vi "SWaT pump flow.vi"(4 "State":i16, 5 "Time":dbl format="%.2f", 6 "Sensor Values":dbl[](array[numeric]), 7 "Set Points":dbl[](array[numeric])) -> (0 "required data":T1={"Set Point names"=["L Tube Settler (mm)", "D Tube Settler (mm)", "Tube angle (degrees)", "Capture Velocity (mm/s)", ""], "required number of setpoints"=4, "required number of sensors"=0, "Sensor names"=[]}, 3 "output value":dbl)   [LabVIEW 2019]
panel:
  # "Enter the correct information for this control code in the required data structure below. Then make the current value default by right clicking on the border of the data structure."
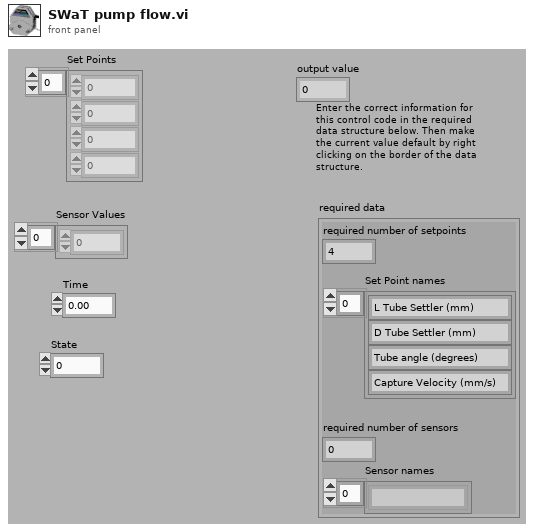
[diagram p1: front panel]
types:
  T1 = cluster{"Set Point names":string[], "required number of setpoints":u8, "required number of sensors":u8, "Sensor names":string[]}
  T2 = cluster{"Set Points[0]":dbl, "Set Points[1]":dbl, "Set Points[2]":dbl, "Set Points[3]":dbl, "Set Points[4]":dbl}
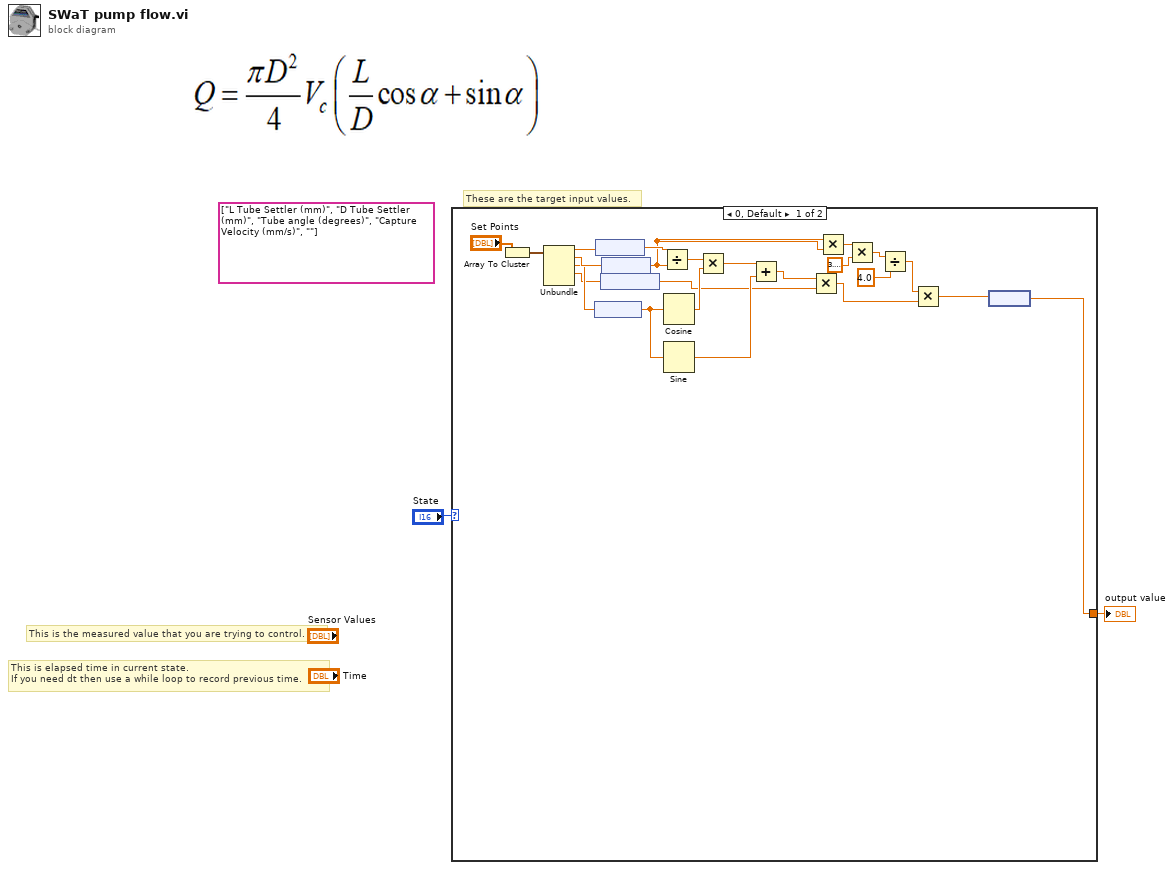
[diagram p0: block diagram]
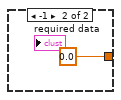
[diagram p2: hidden frame]
diagram:
  (unwired) string[] ["L Tube Settler (mm)", "D Tube Settler (mm)", "Tube angle (degrees)", "Capture Velocity (mm/s)", ""] ("Set Point names")
  # "These are the target input values."
  # "This is the measured value that you are trying to control."
  # "This is elapsed time in current state.\nIf you need dt then use a while loop to record previous time."
  n1 = case shown="0, Default" "State" {
    tunnel: [w7 0.0 ("fraction on")] -> w1
    frame 0, Default {
      n2 = Array To Cluster(array="Set Points") -> (cluster=w25:T2)
      n3 = Unbundle(w25) -> ("Set Points[0]"=w6:dbl, "Set Points[1]"=w5:dbl, "Set Points[2]"=w4:dbl, "Set Points[3]"=w3:dbl)  [unwired: 1 out]
      n4 = node(w4) -> (w14:dbl[unit])
      n5 = node(w6) -> (w10:dbl[unit])
      n6 = node(w3) -> (w13:dbl[unit])
      n7 = node(w5) -> (w9:dbl[unit])
      n8 = Divide(x=w10, y=w9) -> (x/y=w23:dbl)
      n9 = Cosine(x=w14) -> (cos(x)=w22:dbl)
      n10 = Sine(x=w14) -> (sin(x)=w20:dbl)
      n11 = Multiply(x=w23, y=w22) -> (x*y=w21:dbl)
      n12 = Add(x=w21, y=w20) -> (x+y=w19:dbl)
      n13 = Multiply(x=w19, y=w13) -> (x*y=w11:dbl[unit])
      n14 = Multiply(x=w9, y=w9) -> (x*y=w18:dbl[unit])
      n15 = Multiply(x=w18, y=3.141592653589793) -> (x*y=w16:dbl[unit])
      n16 = Divide(x=w16, y=4.0) -> (x/y=w12:dbl[unit])
      n17 = Multiply(x=w12, y=w11) -> (x*y=w8:dbl[unit])
      n18 = node(w8) -> (w7:dbl)
    }
    frame -1 {
    }
  }
  "output value" <- w1
